vi "message_deliver.vi"(0 "communication type":enum16{"SV", "Dim"}(ring), 1 "shared variable refnum":refnum<k21>, 3 "MoAgSy_Message":refnum<class "MoAgSy_Message.lvclass">, 5 "error in (no error)":errorcluster) -> (19 "error out":errorcluster)   [LabVIEW 2009, in "MoAgSy.lvlib" / "MoAgSy_Host.lvclass"]
doc: "<B>public</B> VI delivers a message.\nMessage will be flattened to string and wrote to SV.\n<B>in progress\nnot implemented Yet:\nDIM support\nGPG support\n</B>\nF.Berck@gsi.de\nGSI Darmstadt 2009"
uses:
  MoAgSy_Host.lvclass
  MoAgSy_Message/MoAgSy_Message.lvclass
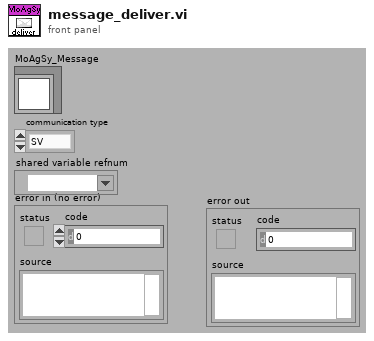
[diagram p1: front panel]
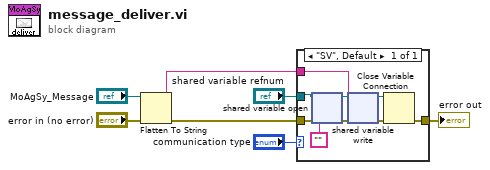
[diagram p0: block diagram]
diagram:
  n1 = Flatten To String(anything="MoAgSy_Message", error in (no error)="error in (no error)") -> (data string=w4:string, error out=w3:errorcluster)  [unwired: 3 out]
  n2 = case shown="\"SV\", Default" "communication type" {
    tunnel: w4 -> [w11]
    tunnel: w3 -> [w15]
    tunnel: "shared variable refnum" -> [w16]
    tunnel: [w8] -> w1
    frame "SV", Default {
      n3 = shared-variable-open(w16, w15, "") -> (w13:refnum<k21>, w12:errorcluster)  [unwired: 1 in]
      n4 = shared-variable-write(w13, w12, w11) -> (w9:refnum<k21>, w10:errorcluster)
      n5 = Close Variable Connection(8:w10, 11:w9) -> (0:w8:errorcluster)
    }
  }
  "error out" <- w1
